vi "BezierGeneratorRev2.vi"(1 "RobotY":dbl, 2 "RobotX":dbl, 3 "DeltaYaw":dbl, 4 "RobotOrientation":dbl=70.0, 5 "DeltaY":dbl=60.0, 6 "DeltaX":dbl=60.0) -> (0 "RobotNeededPathData":T1={"Path"=[], "MaxVel"=80.0, "MaxAccel"=100.0, "Backwards?"=FALSE, "PointSpacing"=6.0, "LookaheadDist"=13.0, "Speed/Curve"=1.8, "SlowDistanceAtEnd"=0.0, "SlowSpeed"=0.0, "MaxDeAccel"=80.0} {"SlowSpeed" format="%#_13g"; "SlowDistanceAtEnd" format="%#_13g"; "Speed/Curve" format="%#_13g"})   [LabVIEW 2018]
uses:
  Dawgma-Programming-Library-master/Dawgma-Programming-Library-master/Controls/PurePursuit/RobotNeededPathData.ctl
panel:
  in  "SlowSpeed":dbl
  in  "SlowDistanceAtEnd":dbl
  in  "Speed/Curve":dbl=1.8
  in  "LookaheadDist":dbl=13.0
  in  "PointSpacing":dbl=6.0
  in  "MaxDeaccel":dbl=80.0
  in  "MaxAccel":dbl=100.0
  in  "MaxVel":dbl=80.0
  out "Curve":cluster{"X":dbl, "Y":dbl}[](graph)
  out "waypoints":cluster{dbl[], dbl[]}(graph)
  in  "TrajPointoffset":dbl=12.0
  in  "TargetOffset":dbl=12.0
  in  "Path":cluster{"x":dbl, "y":dbl}[](array[cluster])=[{"x"=0.0, "y"=0.0}, {"x"=0.0, "y"=0.0}, {"x"=0.0, "y"=0.0}, {"x"=0.0, "y"=0.0}]
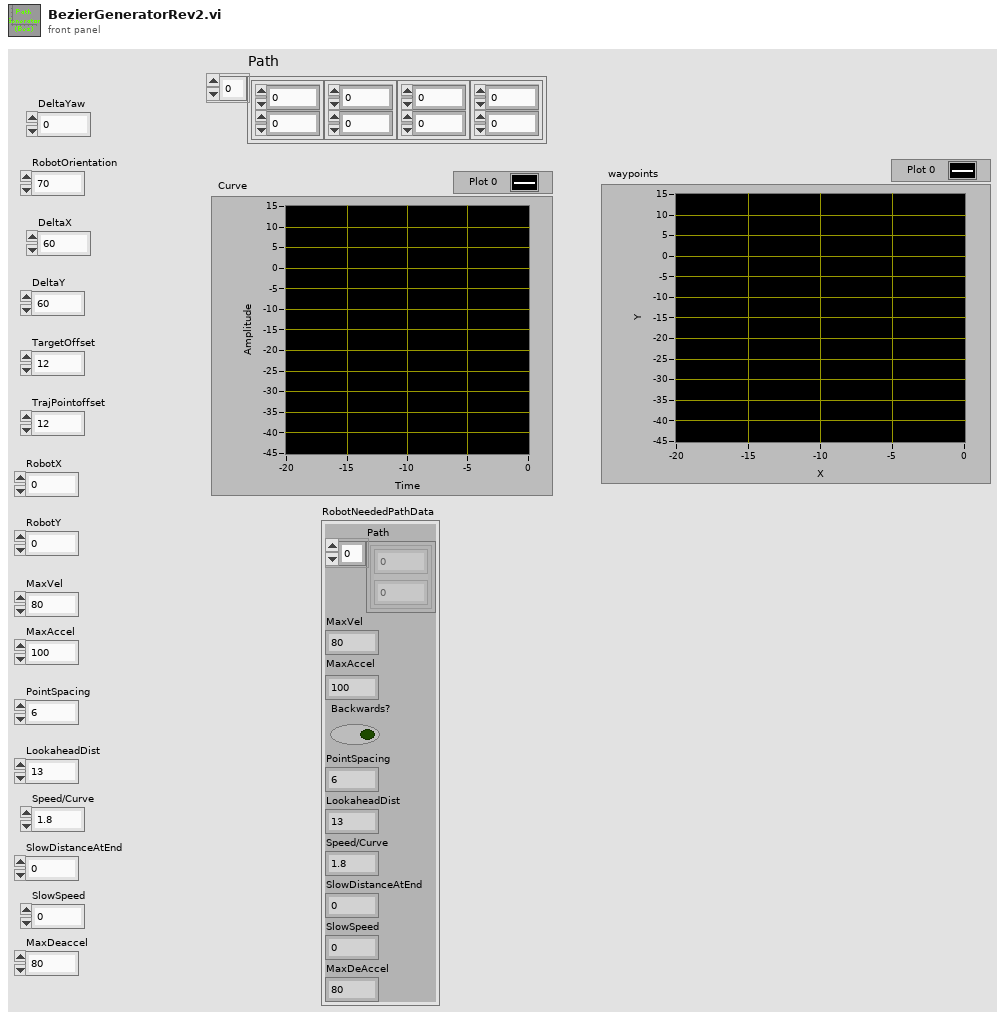
[diagram p1: front panel]
types:
  T1 = typedef "RobotNeededPathData.ctl" = cluster{"Path":cluster{dbl, dbl}[], "MaxVel":dbl, "MaxAccel":dbl, "Backwards?":bool, "PointSpacing":dbl, "LookaheadDist":dbl, "Speed/Curve":dbl, "SlowDistanceAtEnd":dbl, "SlowSpeed":dbl, "MaxDeAccel":dbl}
  T2 = cluster{"DeltaX":dbl, "DeltaY":dbl, "RobotOrientation":dbl, "TrajPointoffset":dbl, "TargetOffset":dbl}
  T3 = cluster{cluster{"x":dbl, "y":dbl}[], "MaxVel":dbl, "MaxAccel":dbl, bool, "PointSpacing":dbl, "LookaheadDist":dbl, "Speed/Curve":dbl, "SlowDistanceAtEnd":dbl, "SlowSpeed":dbl, "MaxDeaccel":dbl}
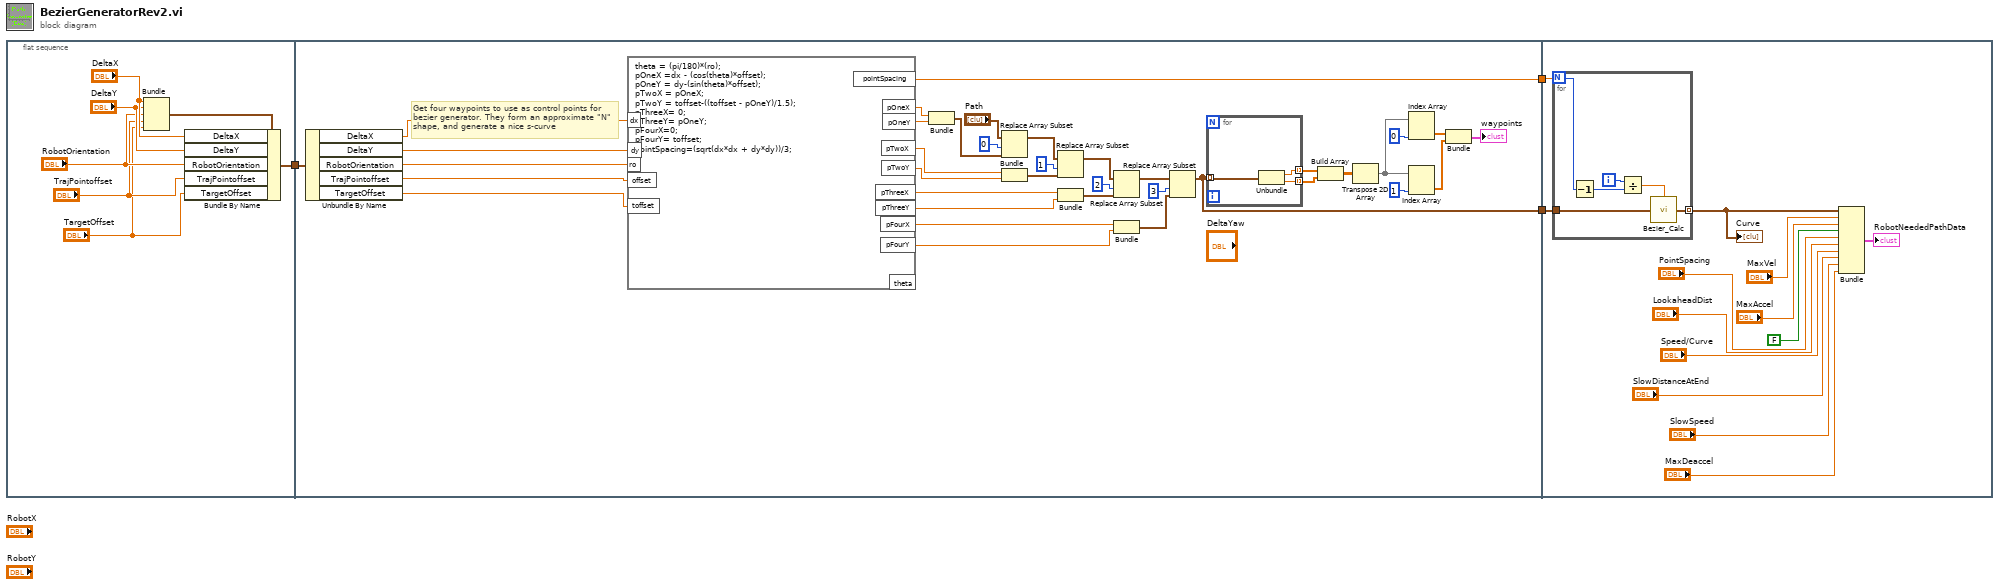
[diagram p0: block diagram]
diagram:
  n1 = flat-sequence {
    tunnel: [w9] -> w1
    tunnel: [w29] -> w3
    tunnel: [w17] -> w2
    tunnel: w1 -> [w23]
    tunnel: w3 -> [w63]
    tunnel: w2 -> [w62]
    frame #0 {
      n2 = Bundle("DeltaX"="DeltaX", "DeltaY"="DeltaY", "RobotOrientation"="RobotOrientation", "TrajPointoffset"="TrajPointoffset", "TargetOffset"="TargetOffset") -> (w10:T2)  [unwired: 1 in]
      n3 = Bundle By Name(cluster=w10, "DeltaX"="DeltaX", "DeltaY"="DeltaY", "RobotOrientation"="RobotOrientation", "TrajPointoffset"="TrajPointoffset", "TargetOffset"="TargetOffset") -> (w9:T2)
    }
    frame #1 {
      # "Get four waypoints to use as control points for bezier generator. They form an approximate \"N\" shape, and generate a nice s-curve"
      n4 = Unbundle By Name(w23) -> ("DeltaX"=w22:dbl, "DeltaY"=w21:dbl, "RobotOrientation"=w18:dbl, "TrajPointoffset"=w19:dbl, "TargetOffset"=w20:dbl)
      n5 = formula code="theta = (pi/180)*(ro);\npOneX =dx - (cos(theta)*offset);\npOneY = dy-(sin(theta)*offset);\npTwoX = pOneX;\npTwoY = toffset-((toffset - pOneY)/1.5);\npThreeX= 0;\npThreeY= pOneY;\npFourX=0;\npFourY= toffset;\npointSpacing=(sqrt(dx*dx + dy*dy))/3;"("ro"=w18, "dx"=w22, "dy"=w21, "offset"=w19, "toffset"=w20) -> ("pOneX"=w27:dbl, "pOneY"=w26:dbl, "pTwoX"=w25:dbl, "pTwoY"=w24:dbl, "pointSpacing"=w17:dbl, "pThreeX"=w16:dbl, "pThreeY"=w15:dbl, "pFourX"=w14:dbl, "pFourY"=w13:dbl)  [unwired: 1 out]
      n6 = Bundle("pOneX"=w27, "pOneY"=w26) -> (w38:cluster{"pOneX":dbl, "pOneY":dbl})  [unwired: 1 in]
      n7 = Replace Array Subset(array="Path", new element=w38, index=0) -> (w44:cluster{"x":dbl, "y":dbl}[])
      n8 = Bundle("pTwoX"=w25, "pTwoY"=w24) -> (w39:cluster{"pTwoX":dbl, "pTwoY":dbl})  [unwired: 1 in]
      n9 = Replace Array Subset(array=w44, new element=w39, index=1) -> (w42:cluster{"x":dbl, "y":dbl}[])
      n10 = Bundle("pThreeX"=w16, "pThreeY"=w15) -> (w11:cluster{"pThreeX":dbl, "pThreeY":dbl})  [unwired: 1 in]
      n11 = Replace Array Subset(array=w42, new element=w11, index=2) -> (w40:cluster{"x":dbl, "y":dbl}[])
      n12 = Bundle("pFourX"=w14, "pFourY"=w13) -> (w12:cluster{"pFourX":dbl, "pFourY":dbl})  [unwired: 1 in]
      n13 = Replace Array Subset(array=w40, new element=w12, index=3) -> (w29:cluster{"x":dbl, "y":dbl}[])
      n14 = for {
        tunnel: w29 -> [w50] mode=indexing
        tunnel: [w49] -> w37 mode=indexing
        tunnel: [w48] -> w36 mode=indexing
        n15 = Unbundle(w50) -> ("x"=w49:dbl, "y"=w48:dbl)
      }
      n16 = Build Array(w37, w36) -> (w35:dbl[][])
      n17 = Transpose 2D Array(2D array=w35) -> (transposed array=w32:dbl[][])
      n18 = Index Array(array=w32, index (col)=0 ("disabled index (col)")) -> (element=w30:dbl[])  [unwired: 1 in]
      n19 = Index Array(array=w32, index (col)=1 ("disabled index (col)")) -> (element=w31:dbl[])  [unwired: 1 in]
      n20 = Bundle(w30, w31) -> (→"waypoints":cluster{dbl[], dbl[]})  [unwired: 1 in]
    }
    frame #2 {
      n21 = for {
        N: w62 -> [w69]
        tunnel: w63 -> [w65]
        tunnel: [w64] -> w61 mode=indexing
        i -> [w68]
        n22 = Decrement(x=w69) -> (x-1=w67:i32)
        n23 = Divide(x=w68, y=w67) -> (x/y=w66:dbl)
        n24 = call "Bezier_Calc.vi"("points"=w65, "t"=w66) -> ("point out"=w64:cluster{"x":dbl, "y":dbl})
      }
      "Curve" <- w61
      n25 = Bundle(w61, "MaxVel"="MaxVel", "MaxAccel"="MaxAccel", FALSE, "PointSpacing"="PointSpacing", "LookaheadDist"="LookaheadDist", "Speed/Curve"="Speed/Curve", "SlowDistanceAtEnd"="SlowDistanceAtEnd", "SlowSpeed"="SlowSpeed", "MaxDeaccel"="MaxDeaccel") -> (→"RobotNeededPathData":T3)  [unwired: 1 in]
    }
  }
